vi "Log.vi"(8 "error in (no error)":errorcluster, 10 "LogRecord":refnum<class "LogRecord.lvclass">, 11 "NetworkHandler in":refnum<class "StreamLogHandle.lvclass">) -> (0 "error out":errorcluster, 3 "NetworkHandler out":refnum<class "StreamLogHandle.lvclass">)   [LabVIEW 2024, in "StreamLogHandle.lvclass"]
uses:
  StreamLogHandle.lvclass
  Record/LogRecord.lvclass
  StreamLogHandle.lvclass/StreamLogHandle.ctl
  <vilib>/Utility/error.llb/Trim Whitespace One-Sided.vi
  Stream/INetworkWriter/INetworkWriter.lvclass
  LogFormatter/Interface/ILogFormatter.lvclass
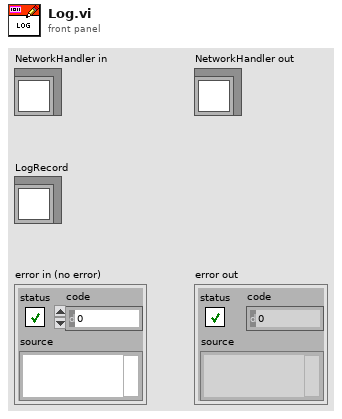
[diagram p1: front panel]
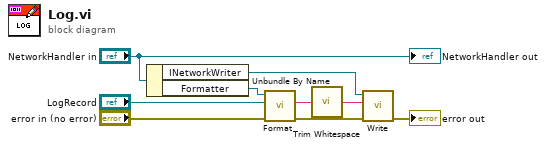
[diagram p0: block diagram]
diagram:
  n1 = Unbundle By Name("NetworkHandler in") -> ("INetworkWriter"=w6:refnum<class "INetworkWriter.lvclass">, "Formatter"=w8:refnum<class "ILogFormatter.lvclass">)
  n2 = call-dynamic "Format.vi"("error in (no error)"="error in (no error)", "LogRecord"="LogRecord", "ILogFormatter in"=w8) -> ("error out"=w4:errorcluster, "Log Line"=w5:string)  [unwired: 6 in, 1 out]
  n3 = call <vilib>:"Trim Whitespace.vi"("string"=w5) -> ("trimmed string"=w1:string)  [unwired: 1 in]
  n4 = call-dynamic "Write.vi"("error in (no error)"=w4, "Message"=w1, "INetworkWriter in"=w6) -> ("error out"=→"error out":errorcluster)  [unwired: 7 in, 1 out]
  "NetworkHandler out" <- "NetworkHandler in"
